vi "DisableControls.vi"(0 "Array":refnum<vi>[](array[refnum]), 1 "User Input":T1(ring)=enum."Disabled", 2 "Menu action":T1(ring), 3 "Card Simulator":T1(ring)=enum."Disabled", 11 "Error In":errorcluster) -> (15 "Error Out":errorcluster)   [LabVIEW 2017]
doc: "This VI is responsible foe enabling and disabling of the controls and indicators present on FP based on the user selection."
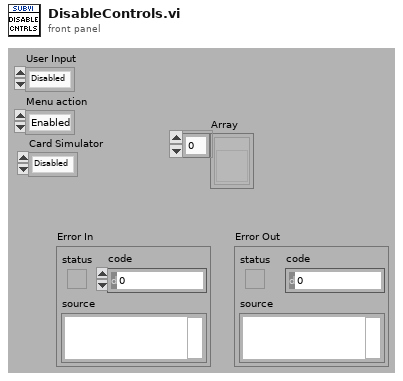
[diagram p1: front panel]
types:
  T1 = enum8{"Enabled", "Disabled", "Disabled and Grayed Out"}
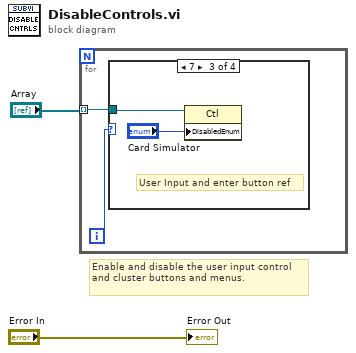
[diagram p0: block diagram]
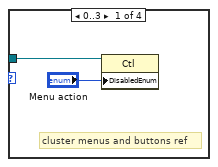
[diagram p2: hidden frame]
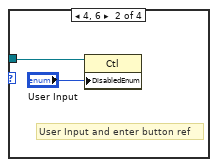
[diagram p3: hidden frame]
diagram:
  # "Enable and disable the user input control\nand cluster buttons and menus."
  n1 = for {
    tunnel: "Array" -> [w4] mode=indexing
    i -> [w3]
    n2 = case shown="7" w3 {
      tunnel: w4 -> [w6 w8 w10 _]
      frame 0..3 {
        # "cluster menus and buttons ref"
        n3 = property class="Ctl"(reference=w6, "DisabledEnum"="Menu action") -> ()  [unwired: 1 in, 2 out]
      }
      frame 4, 6 {
        # "User Input and enter button ref"
        n4 = property class="Ctl"(reference=w8, "DisabledEnum"="User Input") -> ()  [unwired: 1 in, 2 out]
      }
      frame 7 {
        # "User Input and enter button ref"
        n5 = property class="Ctl"(reference=w10, "DisabledEnum"="Card Simulator") -> ()  [unwired: 1 in, 2 out]
      }
      frame Default {
      }
    }
  }
  "Error Out" <- "Error In"
